vi "filter_logic_delays2.vi"(9 "Filter Limits":T2, 10 "Variables Cluster":T4, 11 "Limits Cluster":T1={"High Charge Limit"=0, "Low Charge Limit"=0, "Time Out Limit"=0, "High Velocity Count"=0, "Low Velocity Count"=0, "Sampling Rate"=26666666.59375, "High Mass Limit"=0, "Low Mass Limit"=0}) -> (3 "Output Cluster":T3)   [LabVIEW 2015]
uses:
  Filter Logic In.ctl
  Filter Cutoffs.ctl
  Limits.ctl
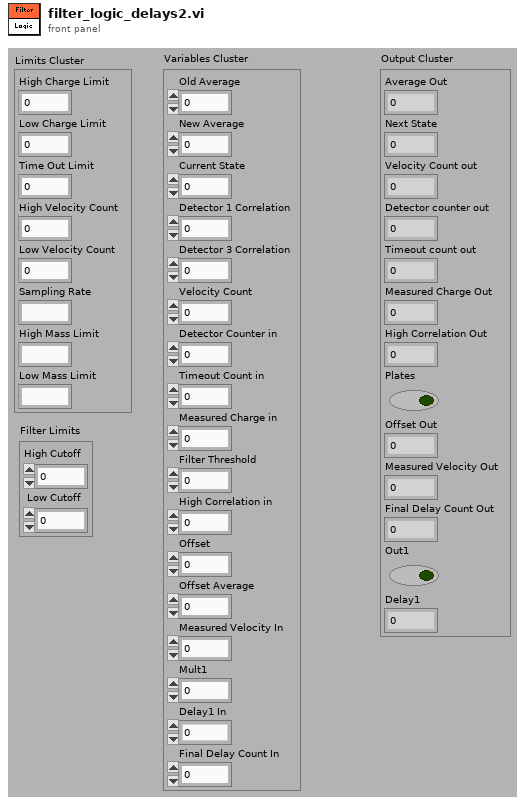
[diagram p1: front panel]
types:
  T1 = typedef "Limits.ctl" = cluster{"High Charge Limit":i16, "Low Charge Limit":i16, "Time Out Limit":i32, "High Velocity Count":i32, "Low Velocity Count":i32, "Sampling Rate":fxp<+,30,25>, "High Mass Limit":i64, "Low Mass Limit":i64}
  T2 = typedef "Filter Cutoffs.ctl" = cluster{"High Cutoff":i32, "Low Cutoff":i32}
  T3 = cluster{"Average Out":i32, "Next State":u8, "Velocity Count out":i32, "Detector counter out":i32, "Timeout count out":u32, "Measured Charge Out":i32, "High Correlation Out":i32, "Plates":bool, "Offset Out":i32, "Measured Velocity Out":i32, "Final Delay Count Out":u16, "Out1":bool, "Delay1":i32}
  T4 = typedef "Filter Logic In.ctl" = cluster{"Old Average":i16, "New Average":i16, "Current State":u8, "Detector 1 Correlation":i16, "Detector 3 Correlation":i16, "Velocity Count":i32, "Detector Counter in":i32, "Timeout Count in":u32, "Measured Charge in":i32, "Filter Threshold":i32, "High Correlation in":i32, "Offset":i32, "Offset Average":i32, "Measured Velocity In":i32, "Mult1":fxp<+,16,7>, "Delay1 In":i32, "Final Delay Count In":u16}
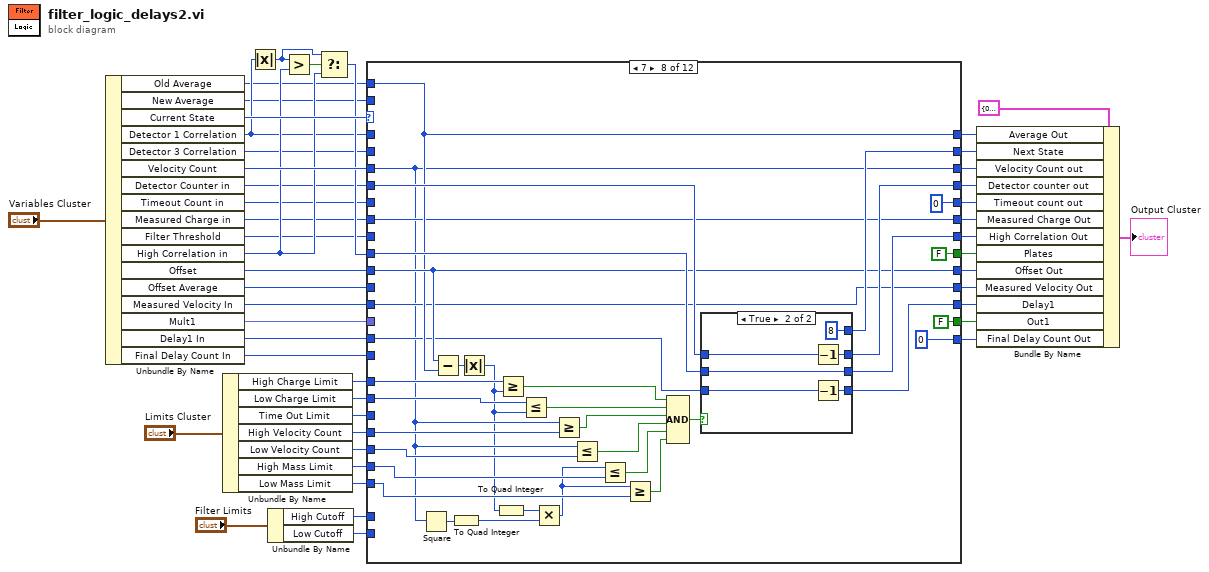
[diagram p0: block diagram]
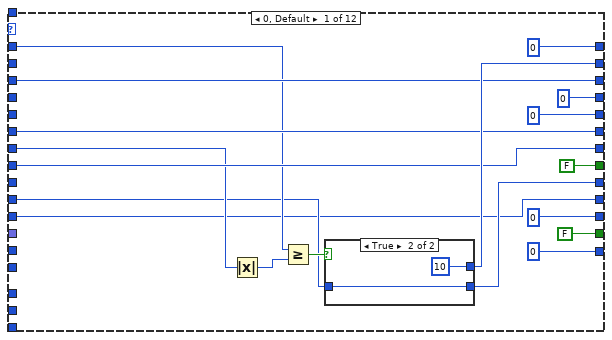
[diagram p2: hidden frame]
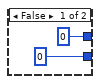
[diagram p3: hidden frame]
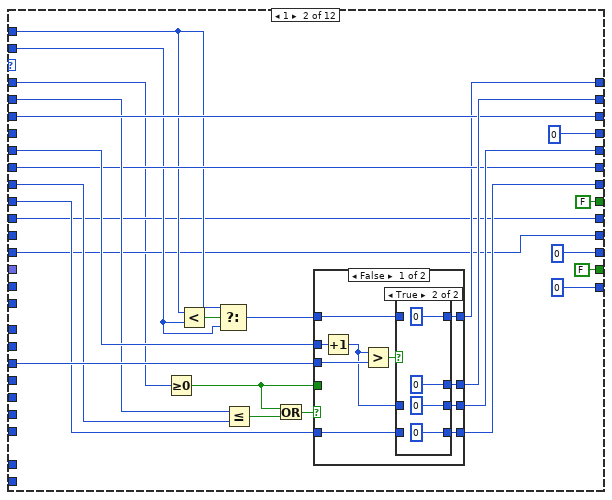
[diagram p4: hidden frame]
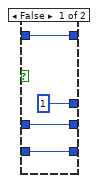
[diagram p5: hidden frame]
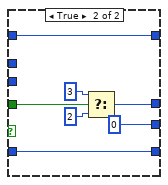
[diagram p6: hidden frame]
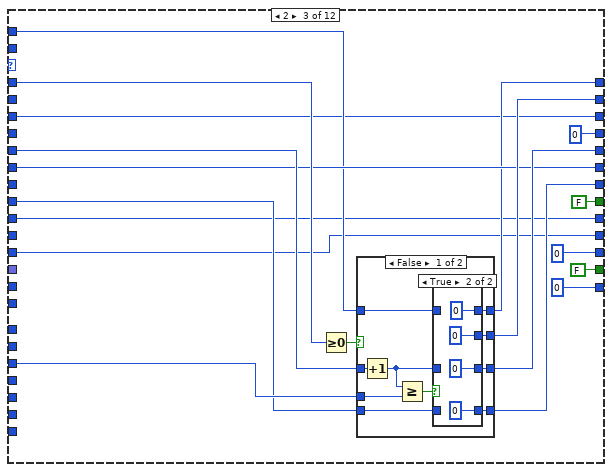
[diagram p7: hidden frame]
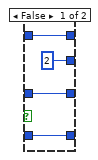
[diagram p8: hidden frame]
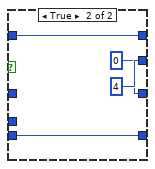
[diagram p9: hidden frame]
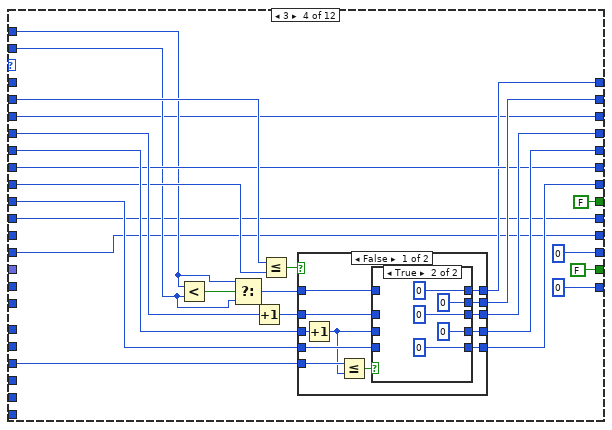
[diagram p10: hidden frame]
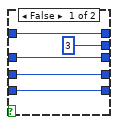
[diagram p11: hidden frame]
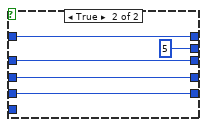
[diagram p12: hidden frame]
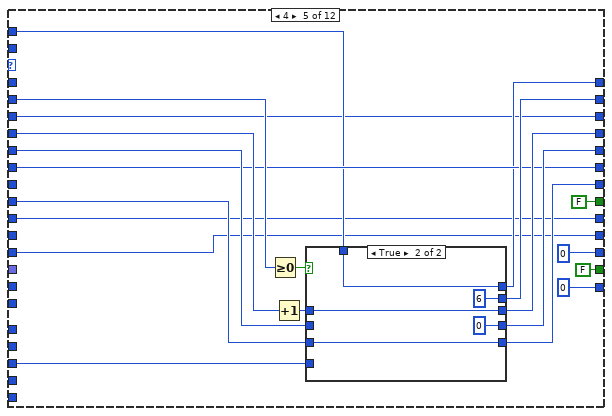
[diagram p13: hidden frame]
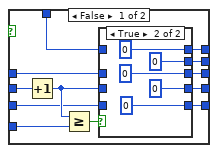
[diagram p14: hidden frame]
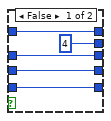
[diagram p15: hidden frame]
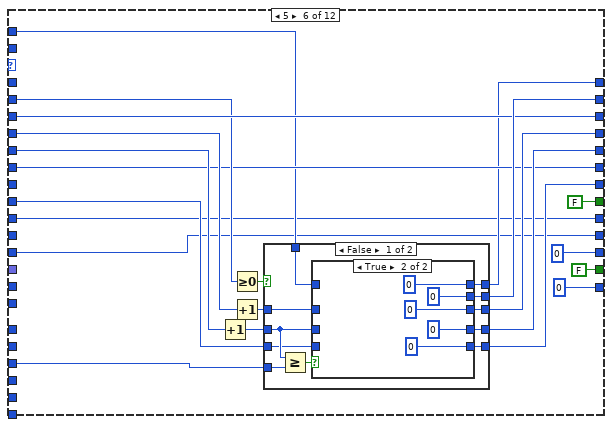
[diagram p16: hidden frame]
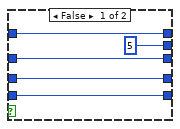
[diagram p17: hidden frame]
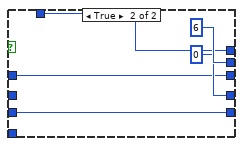
[diagram p18: hidden frame]
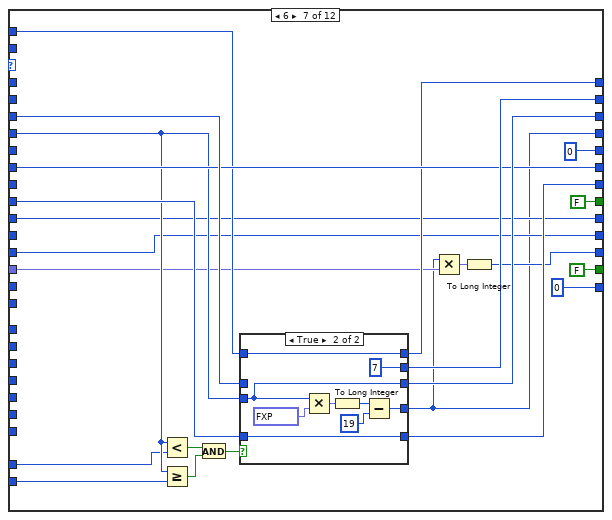
[diagram p19: hidden frame]
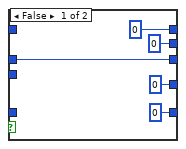
[diagram p20: hidden frame]
diagram:
  n1 = Unbundle By Name("Variables Cluster") -> ("Old Average"=w23:i16, "New Average"=w22:i16, "Current State"=w43:u8, "Detector 1 Correlation"=w33:i16, "Detector 3 Correlation"=w32:i16, "Velocity Count"=w42:i32, "Detector Counter in"=w36:i32, "Timeout Count in"=w35:u32, "Measured Charge in"=w34:i32, "Filter Threshold"=w37:i32, "High Correlation in"=w38:i32, "Offset"=w21:i32, "Offset Average"=w20:i32, "Measured Velocity In"=w17:i32, "Mult1"=w2:fxp<+,16,7>, "Delay1 In"=w5:i32, "Final Delay Count In"=w8:u16)
  n2 = Unbundle By Name("Limits Cluster") -> ("High Charge Limit"=w16:i16, "Low Charge Limit"=w15:i16, "Time Out Limit"=w14:i32, "High Velocity Count"=w13:i32, "Low Velocity Count"=w12:i32, "High Mass Limit"=w11:i64, "Low Mass Limit"=w10:i64)
  n3 = Absolute Value(x=w33) -> (abs(x)=w39:i16)
  n4 = Unbundle By Name("Filter Limits") -> ("High Cutoff"=w46:i32, "Low Cutoff"=w45:i32)
  n5 = Greater?(x=w39, y=w38) -> (0:w40:bool)
  n6 = Select(t=w39, s=w40, f=w38) -> (s? t:f=w41:i32)
  n7 = case shown="7" w43 {
    tunnel: w33 -> [w58 w70 w135 _ _ _ _ _ _ _ w469 _]
    tunnel: w32 -> [_ w87 _ w178 w226 w273 _ _ _ _ _ _]
    tunnel: w37 -> [w56 w86 _ w177 _ _ _ _ _ _ w468 _]
    tunnel: w36 -> [_ _ _ w180 w234 w282 w325 w382 w411 w441 _ _]
    tunnel: [0 0 0 w186 w232 w275 w310 w381 w409 w439 0 0] -> w29
    tunnel: [w65 w95 w139 w185 w229 w278 w330 w380 w410 w440 w466 w504] -> w25
    tunnel: w42 -> [w62 w88 w126 w166 w218 w274 w331 w356 w395 w437 w461 w495]
    tunnel: w14 -> [_ w94 w138 w183 w227 w279 _ _ _ _ w464 _]
    tunnel: w35 -> [_ w93 w137 w184 w228 w281 _ _ _ _ w465 _]
    tunnel: [u32 0 w92 w136 w182 w230 w277 u32 0 u32 0 ("Timeout Count in") u32 0 ("Timeout Count in") u32 0 w456 u32 0 ("Timeout Count in")] -> w28
    tunnel: w12 -> [_ _ _ _ _ _ _ w379 _ _ _ _]
    tunnel: w13 -> [_ _ _ _ _ _ _ w378 _ _ _ _]
    tunnel: [w62 w88 w126 w166 w218 w274 w332 w356 w395 w437 w461 w495] -> w31
    tunnel: w15 -> [_ _ _ _ _ _ _ w377 _ _ _ _]
    tunnel: w16 -> [_ _ _ _ _ _ _ w376 _ _ _ _]
    tunnel: w41 -> [w61 w85 w133 w176 w221 w272 w328 w375 w407 w435 w458 _]
    tunnel: [w61 w84 w132 w175 w225 w271 w329 w374 w407 w436 w458 0 ("Noise Level")] -> w26
    tunnel: w34 -> [w60 w83 w131 w174 w224 w270 w327 w357 w403 w432 w459 w497]
    tunnel: [w60 w83 w131 w174 w224 w270 w327 w357 w404 w432 w459 w497] -> w27
    tunnel: [0 ("Old Average In") w82 w130 w173 w223 w269 w326 w370 w400 0 ("Old Average In") w462 0 ("Old Average In")] -> w30
    tunnel: w46 -> [_ _ _ _ _ _ w312 _ _ _ _ _]
    tunnel: w45 -> [_ _ _ _ _ _ w311 _ _ _ _ _]
    tunnel: [FALSE FALSE FALSE FALSE FALSE FALSE FALSE FALSE ("Data") w394 w426 FALSE ("Data") FALSE ("Data")] -> w24
    tunnel: w23 -> [_ w79 w128 w170 w220 w267 w322 w370 w400 _ w470 _]
    tunnel: w22 -> [_ w78 _ w169 _ _ _ _ _ _ w450 _]
    tunnel: w21 -> [_ w76 w127 w167 w219 w266 w321 w371 w399 _ w455 _]
    tunnel: w20 -> [w53 _ _ _ _ _ _ _ _ _ _ _]
    tunnel: [w54 w76 w127 w167 w219 w266 w321 w371 w399 0 ("Offset") w455 0 ("Offset")] -> w19
    tunnel: [w52 w75 w125 w165 w217 w265 w320 w358 w405 w430 w454 w502] -> w18
    tunnel: w17 -> [w52 w75 w125 w165 w217 w265 w320 w358 w406 w430 w454 w502]
    tunnel: w11 -> [_ _ _ _ _ _ _ w369 _ _ _ _]
    tunnel: w10 -> [_ _ _ _ _ _ _ w368 _ _ _ _]
    tunnel: w5 -> [_ _ _ _ _ _ _ w364 w398 w429 _ w493]
    tunnel: [0 0 0 0 0 0 w316 w363 w396 w424 0 w490] -> w6
    tunnel: [FALSE FALSE FALSE FALSE FALSE FALSE FALSE FALSE w393 w425 FALSE w494] -> w7
    tunnel: [u16 0 u16 0 u16 0 u16 0 u16 0 u16 0 u16 0 u16 0 u16 0 w428 u16 0 w503] -> w9
    tunnel: w8 -> [_ _ _ _ _ _ _ _ _ _ _ w491]
    tunnel: w2 -> [_ _ _ _ _ _ w315 _ _ _ _ _]
    frame 0, Default {
      n8 = Absolute Value(x=w56) -> (abs(x)=w55:i32)
      n9 = Greater Or Equal?(x=w58, y=w55) -> (x >= y?=w63:bool)
      n10 = case shown="True" w63 {
        tunnel: [u8 0 u8 10] -> w65
        tunnel: [0 w68] -> w54
        tunnel: w53 -> [_ w68]
        frame False {
        }
        frame True {
        }
      }
    }
    frame 1 {
      n11 = Greater Or Equal To 0?(x=w70) -> (x >= 0?=w90:bool)
      n12 = Less?(x=w79, y=w78) -> (x < y?=w80:bool)
      n13 = Select(t=w79, s=w80, f=w78) -> (s? t:f=w77:i16)
      n14 = Less Or Equal?(x=w87, y=w86) -> (x <= y?=w89:bool)
      n15 = Or(x=w90, y=w89) -> (x .or. y?=w91:bool)
      n16 = case shown="False" w91 {
        tunnel: [w103 w114] -> w95
        tunnel: w94 -> [w105 _]
        tunnel: w93 -> [w102 _]
        tunnel: [w101 u32 0] -> w92
        tunnel: w90 -> [_ w115]
        tunnel: w85 -> [w100 w119]
        tunnel: [w99 w119] -> w84
        tunnel: [w98 w120] -> w82
        tunnel: w77 -> [w96 w120]
        frame False {
          n17 = Increment(x=w102) -> (x+1=w97:u32)
          n18 = Greater?(x=w97, y=w105) -> (0:w104:bool)
          n19 = case shown="True" w104 {
            tunnel: [u8 1 u8 0 ("Old Average In")] -> w103
            tunnel: w97 -> [w108 _]
            tunnel: [w108 u32 0 ("Old Average In")] -> w101
            tunnel: w100 -> [w107 _]
            tunnel: [w107 0 ("Old Average In")] -> w99
            tunnel: [w106 0 ("Old Average In")] -> w98
            tunnel: w96 -> [w106 _]
            frame False {
            }
            frame True {
            }
          }
        }
        frame True {
          n20 = Select(t=u8 3, s=w115, f=u8 2) -> (s? t:f=w114:u8)
        }
      }
    }
    frame 2 {
      n21 = Greater Or Equal To 0?(x=w135) -> (x >= 0?=w134:bool)
      n22 = case shown="False" w134 {
        tunnel: [w148 u8 4] -> w139
        tunnel: w138 -> [w147 _]
        tunnel: w137 -> [w145 _]
        tunnel: [w146 u32 0] -> w136
        tunnel: w133 -> [w144 w159]
        tunnel: [w143 w159] -> w132
        tunnel: [w142 w158] -> w130
        tunnel: w128 -> [w141 w158]
        frame False {
          n23 = Increment(x=w145) -> (x+1=w140:u32)
          n24 = Greater Or Equal?(x=w140, y=w147) -> (x >= y?=w149:bool)
          n25 = case shown="True" w149 {
            tunnel: [u8 2 u8 0] -> w148
            tunnel: w140 -> [w153 _]
            tunnel: [w153 u32 0] -> w146
            tunnel: w144 -> [w151 _]
            tunnel: [w151 0 ("High Correlation In")] -> w143
            tunnel: [w150 0 ("Old Average In")] -> w142
            tunnel: w141 -> [w150 _]
            frame False {
            }
            frame True {
            }
          }
        }
        frame True {
        }
      }
    }
    frame 3 {
      n26 = Less?(x=w170, y=w169) -> (x < y?=w171:bool)
      n27 = Select(t=w170, s=w171, f=w169) -> (s? t:f=w168:i16)
      n28 = Increment(x=w180) -> (x+1=w179:i32)
      n29 = Less Or Equal?(x=w178, y=w177) -> (x <= y?=w181:bool)
      n30 = case shown="False" w181 {
        tunnel: w179 -> [w194 w213]
        tunnel: [w193 w213] -> w186
        tunnel: [w196 u8 5] -> w185
        tunnel: w184 -> [w192 w209]
        tunnel: w183 -> [w198 _]
        tunnel: [w195 w209] -> w182
        tunnel: w176 -> [w191 w211]
        tunnel: [w190 w211] -> w175
        tunnel: [w189 w210] -> w173
        tunnel: w168 -> [w188 w210]
        frame False {
          n31 = Increment(x=w192) -> (x+1=w187:u32)
          n32 = Less Or Equal?(x=w198, y=w187) -> (x <= y?=w197:bool)
          n33 = case shown="True" w197 {
            tunnel: [u8 3 u8 0] -> w196
            tunnel: w187 -> [w202 _]
            tunnel: [w202 u32 0] -> w195
            tunnel: w194 -> [w201 _]
            tunnel: [w201 0] -> w193
            tunnel: w191 -> [w200 _]
            tunnel: [w200 0 ("High Correlation In")] -> w190
            tunnel: [w199 0 ("Old Average In")] -> w189
            tunnel: w188 -> [w199 _]
            frame False {
            }
            frame True {
            }
          }
        }
        frame True {
        }
      }
    }
    frame 4 {
      n34 = Greater Or Equal To 0?(x=w226) -> (x >= 0?=w233:bool)
      n35 = Increment(x=w234) -> (x+1=w231:i32)
      n36 = case shown="True" w233 {
        tunnel: [w239 w261] -> w232
        tunnel: w231 -> [w240 w261]
        tunnel: [w242 u32 0] -> w230
        tunnel: [w244 u8 6] -> w229
        tunnel: w228 -> [w246 _]
        tunnel: w227 -> [w241 _]
        tunnel: w221 -> [w238 w258]
        tunnel: [w237 w258] -> w225
        tunnel: [w236 w257] -> w223
        tunnel: w220 -> [w235 w257]
        frame False {
          n37 = Increment(x=w246) -> (x+1=w243:u32)
          n38 = Greater Or Equal?(x=w243, y=w241) -> (x >= y?=w245:bool)
          n39 = case shown="True" w245 {
            tunnel: [u8 4 u8 0] -> w244
            tunnel: w243 -> [w250 _]
            tunnel: [w250 u32 0] -> w242
            tunnel: w240 -> [w249 _]
            tunnel: [w249 0] -> w239
            tunnel: w238 -> [w248 _]
            tunnel: [w248 0 ("High Correlation In")] -> w237
            tunnel: [w247 0 ("Old Average In")] -> w236
            tunnel: w235 -> [w247 _]
            frame False {
            }
            frame True {
            }
          }
        }
        frame True {
        }
      }
    }
    frame 5 {
      n40 = Increment(x=w281) -> (x+1=w280:u32)
      n41 = Greater Or Equal To 0?(x=w273) -> (x >= 0?=w283:bool)
      n42 = Increment(x=w282) -> (x+1=w276:i32)
      n43 = case shown="False" w283 {
        tunnel: w280 -> [w290 _]
        tunnel: w279 -> [w294 _]
        tunnel: [w292 u8 6] -> w278
        tunnel: [w291 u32 0] -> w277
        tunnel: w276 -> [w289 w307]
        tunnel: [w288 w307] -> w275
        tunnel: w272 -> [w286 w306]
        tunnel: [w287 w306] -> w271
        tunnel: [w285 w305] -> w269
        tunnel: w267 -> [w284 w305]
        frame False {
          n44 = Greater Or Equal?(x=w290, y=w294) -> (x >= y?=w293:bool)
          n45 = case shown="True" w293 {
            tunnel: [u8 5 u8 0] -> w292
            tunnel: [w298 u32 0] -> w291
            tunnel: w290 -> [w298 _]
            tunnel: w289 -> [w297 _]
            tunnel: [w297 0] -> w288
            tunnel: [w296 0 ("High Correlation In")] -> w287
            tunnel: w286 -> [w296 _]
            tunnel: [w295 0 ("Old Average In")] -> w285
            tunnel: w284 -> [w295 _]
            frame False {
            }
            frame True {
            }
          }
        }
        frame True {
        }
      }
    }
    frame 6 {
      n46 = Less?(x=w325, y=w312) -> (x < y?=w314:bool)
      n47 = Greater Or Equal?(x=w325, y=w311) -> (x >= y?=w313:bool)
      n48 = And(x=w314, y=w313) -> (x .and. y?=w324:bool)
      n49 = case shown="True" w324 {
        tunnel: [0 w342] -> w310
        tunnel: w325 -> [_ w341]
        tunnel: [w338 w341] -> w332
        tunnel: w331 -> [w338 _]
        tunnel: [u8 0 u8 7] -> w330
        tunnel: [0 ("High Correlation In") w346] -> w329
        tunnel: w328 -> [_ w346]
        tunnel: [0 ("Old Average In") w345] -> w326
        tunnel: w322 -> [_ w345]
        frame False {
        }
        frame True {
          n50 = Multiply(x=w341, y=fxp<+,6,1> 1.40625) -> (x*y=w340:fxp<+/-,38,33>)
          n51 = To Long Integer(number=w340) -> (32bit integer=w339:i32)
          n52 = Subtract(x=w339, y=19) -> (x-y=w342:i32)
        }
      }
      n53 = Multiply(x=w310, y=w315) -> (x*y=w318:fxp<+/-,48,39>)
      n54 = To Long Integer(number=w318) -> (32bit integer=w316:i32)
    }
    frame 7 {
      n55 = Square(x=w356) -> (x^2=w352:i32)
      n56 = Subtract(x=w371, y=w370) -> (x-y=w373:i32)
      n57 = To Quad Integer(1:w352) -> (0:w365:i64)
      n58 = Absolute Value(x=w373) -> (abs(x)=w351:i32)
      n59 = To Quad Integer(1:w351) -> (0:w366:i64)
      n60 = Greater Or Equal?(x=w376, y=w351) -> (x >= y?=w355:bool)
      n61 = Less Or Equal?(x=w377, y=w351) -> (x <= y?=w354:bool)
      n62 = Multiply(x=w366, y=w365) -> (x*y=w367:i64)
      n63 = Greater Or Equal?(x=w356, y=w378) -> (x >= y?=w353:bool)
      n64 = Less Or Equal?(x=w356, y=w379) -> (x <= y?=w350:bool)
      n65 = Less Or Equal?(x=w367, y=w369) -> (x <= y?=w348:bool)
      n66 = Greater Or Equal?(x=w367, y=w368) -> (x >= y?=w349:bool)
      n67 = Compound Arithmetic op=AND(w355, w354, w353, w350, w348, w349) -> (w372:bool)
      n68 = case shown="True" w372 {
        tunnel: w382 -> [_ w392]
        tunnel: [0 w390] -> w381
        tunnel: [u8 0 u8 8] -> w380
        tunnel: w375 -> [_ w391]
        tunnel: [0 ("High Correlation In") w391] -> w374
        tunnel: w364 -> [_ w388]
        tunnel: [0 w387] -> w363
        frame False {
        }
        frame True {
          n69 = Decrement(x=w392) -> (x-1=w390:i32)
          n70 = Decrement(x=w388) -> (x-1=w387:i32)
        }
      }
    }
    frame 8 {
      n71 = Decrement(x=w411) -> (x-1=w412:i32)
      n72 = Subtract(x=w399, y=w400) -> (x-y=w402:i32)
      n73 = Less Or Equal To 0?(x=w412) -> (x <= 0?=w394:bool)
      n74 = Absolute Value(x=w402) -> (abs(x)=w401:i32)
      n75 = case shown="True" w394 {
        tunnel: [u8 8 u8 9] -> w410
        tunnel: [w416 w422] -> w409
        tunnel: w395 -> [_ w420]
        tunnel: w412 -> [w416 _]
        tunnel: w406 -> [w414 _]
        tunnel: [w414 w420] -> w405
        tunnel: [w413 w419] -> w404
        tunnel: w403 -> [w413 _]
        tunnel: w401 -> [_ w419]
        frame False {
        }
        frame True {
          n76 = To Fixed-Point(number=w420) -> (fixed-point=w417:fxp<+/-,32,32>)  [unwired: 1 in]
          n77 = Multiply(x=fxp<+,2,1> 1.5, y=w417) -> (x*y=w423:fxp<+/-,34,33>)
          n78 = To Long Integer(number=w423) -> (32bit integer=w422:i32)
        }
      }
      n79 = Decrement(x=w398) -> (x-1=w396:i32)
      n80 = Less Or Equal To 0?(x=w396) -> (x <= 0?=w393:bool)
    }
    frame 9 {
      n81 = Decrement(x=w441) -> (x-1=w438:i32)
      n82 = Less Or Equal To 0?(x=w438) -> (x <= 0?=w427:bool)
      n83 = case shown="False" w427 {
        tunnel: [w444 0] -> w439
        tunnel: [u8 9 u8 12] -> w440
        tunnel: w438 -> [w444 _]
        tunnel: w435 -> [w443 _]
        tunnel: [w443 0 ("Noise Level")] -> w436
        tunnel: [u16 0 u16 550] -> w428
        frame False {
        }
        frame True {
        }
      }
      n84 = Decrement(x=w429) -> (x-1=w424:i32)
      n85 = Not(x=w427) -> (.not. x?=w426:bool)
      n86 = Less Or Equal To 0?(x=w424) -> (x <= 0?=w425:bool)
    }
    frame 10 {
      n87 = Less Or Equal?(x=w469, y=w468) -> (x <= y?=w467:bool)
      n88 = Less?(x=w470, y=w450) -> (x < y?=w471:bool)
      n89 = Select(t=w470, s=w471, f=w450) -> (s? t:f=w463:i16)
      n90 = case shown="False" w467 {
        tunnel: [w477 u8 1] -> w466
        tunnel: w465 -> [w474 _]
        tunnel: w464 -> [w479 _]
        tunnel: w463 -> [w476 _]
        tunnel: [w475 0 ("New Average")] -> w462
        tunnel: [w472 0] -> w456
        frame False {
          n91 = Increment(x=w474) -> (x+1=w473:u32)
          n92 = Greater Or Equal?(x=w473, y=w479) -> (x >= y?=w478:bool)
          n93 = case shown="True" w478 {
            tunnel: [u8 10 u8 0] -> w477
            tunnel: w476 -> [w482 _]
            tunnel: [w482 0 ("New Average")] -> w475
            tunnel: w473 -> [w480 _]
            tunnel: [w480 0] -> w472
            frame False {
            }
            frame True {
            }
          }
        }
        frame True {
        }
      }
    }
    frame 12 {
      n94 = Decrement(x=w493) -> (x-1=w489:i32)
      n95 = Less Or Equal To 0?(x=w489) -> (x <= 0?=w492:bool)
      n96 = case shown="True" w492 {
        tunnel: [FALSE w510] -> w494
        tunnel: [u8 12 w515] -> w504
        tunnel: w491 -> [w508 w516]
        tunnel: [w508 w514] -> w503
        tunnel: [w506 0] -> w490
        tunnel: w489 -> [w506 _]
        frame False {
        }
        frame True {
          n97 = Decrement(x=w516) -> (x-1=w513:u16)
          n98 = Less Or Equal To 0?(x=w513) -> (x <= 0?=w511:bool)
          n99 = case shown="False" w511 {
            tunnel: [u8 12 u8 0] -> w515
            tunnel: [w517 u16 0] -> w514
            tunnel: w513 -> [w517 _]
            frame False {
            }
            frame True {
            }
          }
          n100 = Not(x=w511) -> (.not. x?=w510:bool)
        }
      }
    }
  }
  n101 = Bundle By Name(cluster=T3 {"Average Out"=0, "Next State"=0, "Velocity Count out"=0, "Detector counter out"=0, "Timeout count out"=0, "Measured Charge Out"=0, "High Correlation Out"=0, "Plates"=FALSE, "Offset Out"=0, "Measured Velocity Out"=0, "Final Delay Count Out"=0, "Out1"=FALSE, "Delay1"=0} ("Output Cluster"), "Average Out"=w30, "Next State"=w25, "Velocity Count out"=w31, "Detector counter out"=w29, "Timeout count out"=w28, "Measured Charge Out"=w27, "High Correlation Out"=w26, "Plates"=w24, "Offset Out"=w19, "Measured Velocity Out"=w18, "Delay1"=w6, "Out1"=w7, "Final Delay Count Out"=w9) -> (→"Output Cluster":T3)
